vi "PQconnectPoll.vi"(8 "error in (no error)":errorcluster, 11 "conn":u32) -> (0 "error out":errorcluster, 2 "PollingStatusType":i32, 3 "conn_out":u32)   [LabVIEW 2019, in "libpqlv.lvlib"]
uses:
  libpqlv.lvlib
  libpq.dll
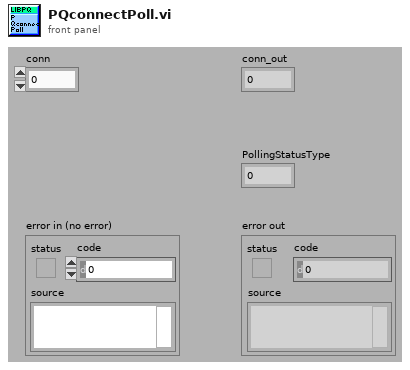
[diagram p1: front panel]
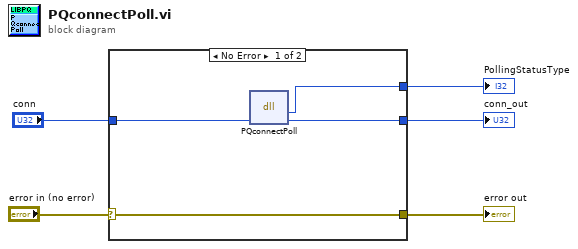
[diagram p0: block diagram]
diagram:
  n1 = case shown="No Error" "error in (no error)" {
    selector: "error in (no error)" -> [w9 w11]
    tunnel: [w9 w11] -> w4
    tunnel: [w8 _] -> w3
    tunnel: [w7 w10] -> w2
    tunnel: "conn" -> [w6 w10]
    frame No Error {
      n2 = dll-call lib="libpq.*" fn="PQconnectPoll"("conn"=w6) -> ("PollingStatusType"=w8:i32, "conn"=w7:u32)  [unwired: 3 in, 2 out]
    }
    frame Error {
    }
  }
  "PollingStatusType" <- w3
  "error out" <- w4
  "conn_out" <- w2
